vi "niRFUtil MT Pack Bits.vi"(0 "input bit stream":i8[](array[numeric]), 5 "bits per integer":i32=1, 7 "packed bit order":enum16{"MSB first", "LSB first"}(ring), 9 "integer format":enum16{"Unsigned", "Signed"}(ring), 11 "error in (no error)":errorcluster, 13 "reset ? (T)":bool=TRUE) -> (4 "output integers":i32[](array[numeric]), 15 "error out":errorcluster)   [LabVIEW 2015, in "niRFUtil.lvlib"]
doc: "Packs data to an unsigned or signed integer array. You can specify the order in which the bits are packed into the integer array either as <B>MSB first</B> or <B>LSB first</B>. You can also specify the integer format to be <B>Signed</B> or <B>Unsigned</B> using the <B>integer format</B> parameter."
uses:
  niRFUtil.lvlib
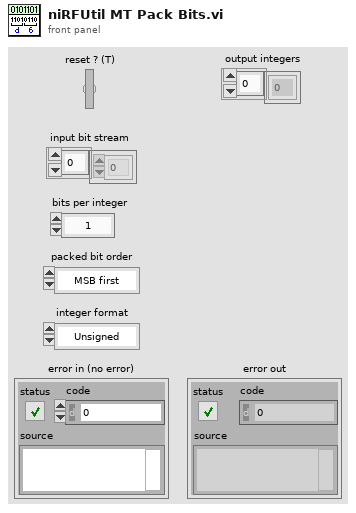
[diagram p1: front panel]
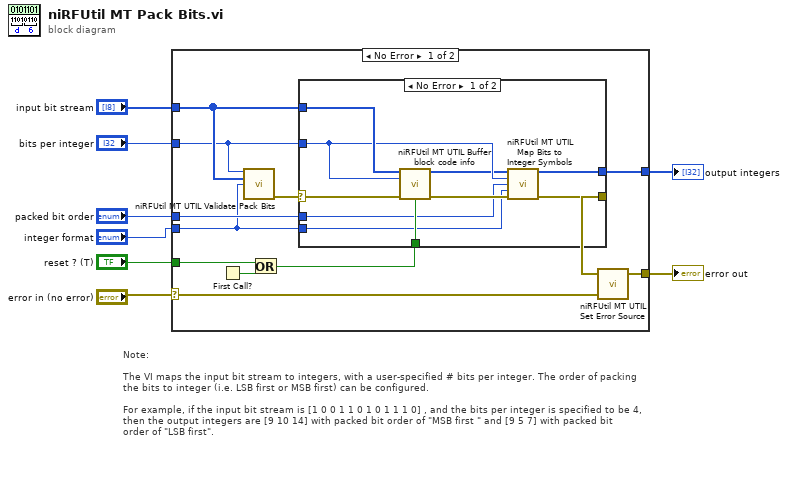
[diagram p0: block diagram]
diagram:
  # "Note:\n\nThe VI maps the input bit stream to integers, with a user-specified # bits per integer. The order of packing\nthe bits to integer (i.e. LSB first or MSB first) can be configured.\n\nFor example, if the input bit stream is [1 0 0 1 1 0 1 0 1 1 1 0] , and the bits per integer is specified to be 4,\nthen the output integers are [9 10 14] with packed bit order of \"MSB first \" and [9 5 7] with packed bit \norder of \"LSB first\"."
  n1 = case shown="No Error" "error in (no error)" {
    selector: "error in (no error)" -> [w12 w32]
    tunnel: "input bit stream" -> [w20 _]
    tunnel: "reset ? (T)" -> [w19 _]
    tunnel: "bits per integer" -> [w16 _]
    tunnel: [w14 _] -> w4
    tunnel: [w11 w32] -> w3
    tunnel: "packed bit order" -> [w10 _]
    tunnel: "integer format" -> [w9 _]
    frame No Error {
      n2 = First Call?() -> (First Call?: T/F=w18:bool)
      n3 = call "niRFUtil MT UTIL Validate Pack Bits.vi"("bits per integer"=w16, "input bit stream"=w20, "integer format"=w9) -> ("error out"=w15:errorcluster)  [unwired: 12 in]
      n4 = Or(x=w19, y=w18) -> (x .or. y?=w17:bool)
      n5 = case shown="No Error" w15 {
        selector: w15 -> [w26 w31]
        tunnel: w20 -> [w27 _]
        tunnel: w17 -> [w30 _]
        tunnel: w16 -> [w24 _]
        tunnel: [w29 w31] -> w13
        tunnel: [w28 _] -> w14
        tunnel: w10 -> [w21 _]
        tunnel: w9 -> [w23 _]
        frame No Error {
          n6 = call "niRFUtil MT UTIL Buffer block code info.vi"("Symbols In"=w27, "Block Size"=w24, "error in (no error)"=w26, "reset? (T)"=w30) -> ("Symbols Out"=w22:i32[], "error out"=w25:errorcluster)  [unwired: 10 in]
          n7 = call "niRFUtil MT UTIL Map Bits to Integer Symbols.vi"("input bit stream"=w22, "bits per integer symbol"=w24, "bit order"=w21, "integer format"=w23, "error in (no error)"=w25) -> ("output integer symbols"=w28:i32[], "error out"=w29:errorcluster)  [unwired: 9 in]
        }
        frame Error {
        }
      }
      n8 = call "niRFUtil MT UTIL Set Error Source.vi"("initial error in (no error)"=w12, "final error in (no error)"=w13) -> ("error out"=w11:errorcluster)  [unwired: 3 in]
    }
    frame Error {
    }
  }
  "error out" <- w3
  "output integers" <- w4
